vi "Write Control Reference.vi"(8 "error in (no error)":errorcluster, 10 "Control Reference":refnum<vi>, 11 "Control Info in":refnum<class "Control Info.lvclass">) -> (0 "error out":errorcluster, 3 "Control Info out":refnum<class "Control Info.lvclass">)   [LabVIEW 2017, in "Localization.lvlib" / "Control Info.lvclass"]
doc: "Writes the Control Reference to the class data.\n\nChoose Movement Consulting, LLC"
uses:
  Control Info.lvclass
  Control Info.lvclass/Control Info.ctl
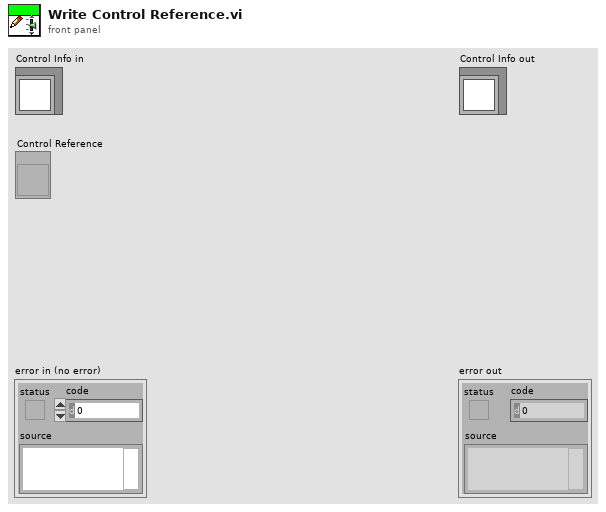
[diagram p1: front panel]
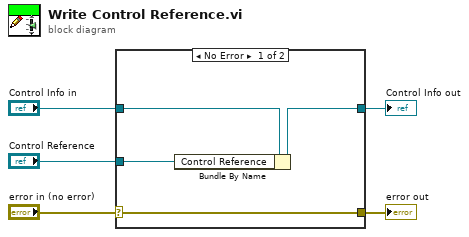
[diagram p0: block diagram]
diagram:
  n1 = case shown="No Error" "error in (no error)" {
    selector: "error in (no error)" -> [w8 w11]
    tunnel: [w8 w11] -> w4
    tunnel: [w7 w10] -> w2
    tunnel: "Control Info in" -> [w9 w10]
    tunnel: "Control Reference" -> [w6 _]
    frame No Error {
      n2 = Bundle By Name(cluster=w9, "Control Reference"=w6) -> (w7:refnum<class "Control Info.lvclass">)
    }
    frame Error {
    }
  }
  "error out" <- w4
  "Control Info out" <- w2
